vi "File_FindCommonRootPath.vi"(1 "Paths":path[](array[path]), 5 "error in (no error)":errorcluster) -> (15 "common root path":path, 17 "Path depth":i32, 19 "error out":errorcluster)   [LabVIEW 2020]
doc: "Finds the common root path of the input path array and returns the common root path and also the nr of levels in the root."
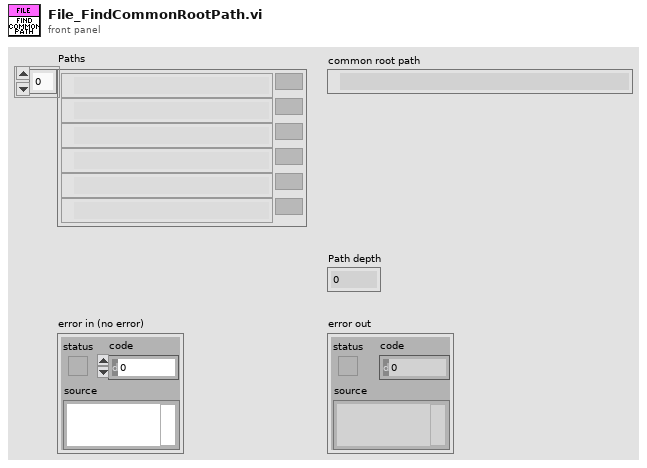
[diagram p1: front panel]
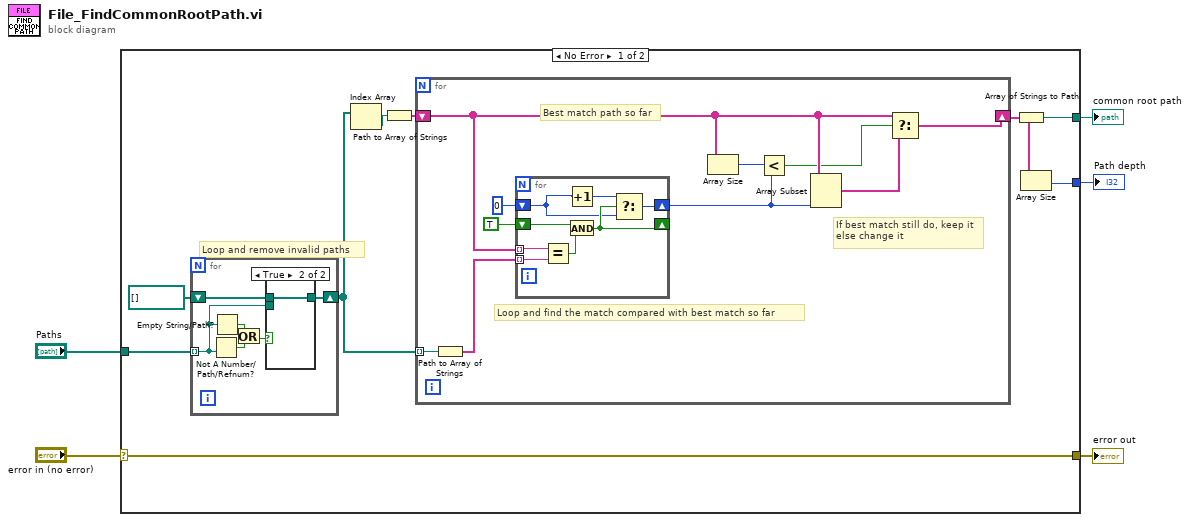
[diagram p0: block diagram]
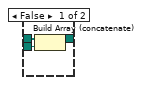
[diagram p2: hidden frame]
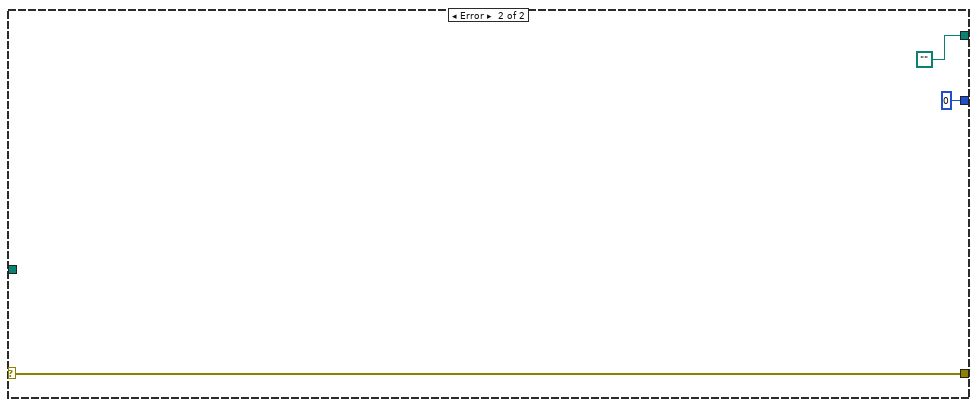
[diagram p3: hidden frame]
diagram:
  n1 = case shown="No Error" "error in (no error)" {
    tunnel: "Paths" -> [w8 _]
    tunnel: [w14 path ""] -> w4
    selector: "error in (no error)" -> [w13 w45]
    tunnel: [w13 w45] -> w2
    tunnel: [w11 0] -> w1
    frame No Error {
      # "Loop and remove invalid paths"
      n2 = for {
        shift-right: [w20] -> w7
        shift-left: path[] [] -> [w18]
        tunnel: w8 -> [w19] mode=indexing
        n3 = Not A Number/Path/Refnum?(number/path/refnum=w19) -> (NaN/Path/Refnum?=w16:bool)
        n4 = Empty String/Path?(string/path=w19) -> (empty?=w17:bool)
        n5 = Or(x=w17, y=w16) -> (x .or. y?=w15:bool)
        n6 = case shown="True" w15 {
          tunnel: [w23 w24] -> w20
          tunnel: w19 -> [w22 _]
          tunnel: w18 -> [w21 w24]
          frame False {
            n7 = Build Array (concatenate)(w21, w22) -> (w23:path[])
          }
          frame True {
          }
        }
      }
      n8 = Index Array(array=w7) -> (element=w10:path)  [unwired: 1 in]
      n9 = Path to Array of Strings(0:w10) -> (2:w9:string[])  [unwired: 1 out]
      n10 = for {
        tunnel: w7 -> [w27] mode=indexing
        shift-right: [w34] -> w12
        shift-left: w9 -> [w28]
        # "If best match still do, keep it\nelse change it"
        # "Best match path so far"
        # "Loop and find the match compared with best match so far"
        n11 = Path to Array of Strings(0:w27) -> (2:w25:string[])  [unwired: 1 out]
        n12 = for {
          tunnel: w28 -> [w42] mode=indexing
          tunnel: w25 -> [w41] mode=indexing
          shift-right: [w38] -> w29
          shift-left: 0 -> [w35]
          shift-right: [w37] -> _
          shift-left: TRUE -> [w39]
          n13 = Equal?(x=w42, y=w41) -> (x = y?=w40:bool)
          n14 = Increment(x=w35) -> (x+1=w36:i32)
          n15 = And(x=w39, y=w40) -> (x .and. y?=w37:bool)
          n16 = Select(t=w36, s=w37, f=w35) -> (s? t:f=w38:i32)
        }
        n17 = Array Size(array=w28) -> (size(s)=w30:i32)
        n18 = Less?(x=w30, y=w29) -> (x < y?=w26:bool)
        n19 = Array Subset(array=w28, length=w29) -> (w33:string[])  [unwired: 1 in]
        n20 = Select(t=w28, s=w26, f=w33) -> (s? t:f=w34:string[])
      }
      n21 = Array of Strings to Path(0:w12) -> (2:w14:path)  [unwired: 1 in]
      n22 = Array Size(array=w12) -> (size(s)=w11:i32)
    }
    frame Error {
    }
  }
  "common root path" <- w4
  "error out" <- w2
  "Path depth" <- w1
